vi "read N samples N channels.vi"(8 "error in (no error)":errorcluster, 11 "DAQ  in":refnum<class "DAQ .lvclass">) -> (0 "error out":errorcluster, 2 "data 2":waveform(dbl)[](array[waveform]), 3 "DAQ  out":refnum<class "DAQ .lvclass">)   [LabVIEW 2017, in "Hardware.lvlib" / "DAQ .lvclass"]
uses:
  DAQ .lvclass
  \\Mac\Home/Documents/MAL-Framework/user.lib/Common Components/Hardware/Hardware.lvclass
  DAQ .lvclass/DAQ .ctl
  MAL-Framework/user.lib/Common Components/Hardware/Hardware.lvclass/Hardware.ctl
  <vilib>/DAQmx/read.llb/DAQmx Read (Analog 1D Wfm NChan NSamp).vi
  <vilib>/DAQmx/miscellaneous.llb/DAQmx Fill In Error Info.vi
  MAL-Framework/user.lib/Common Components/Hardware/Hardware.lvclass
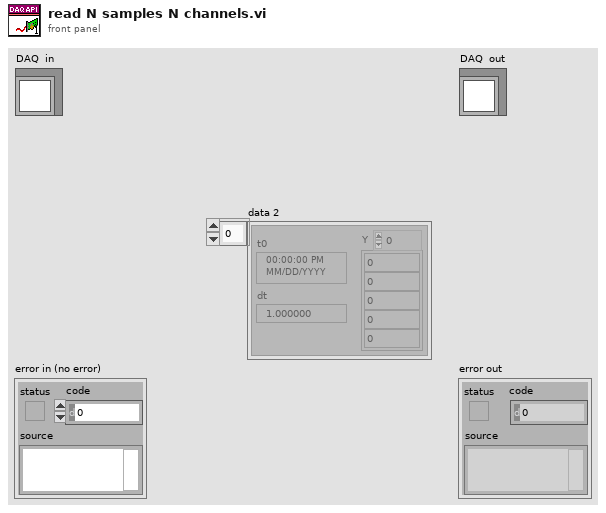
[diagram p1: front panel]
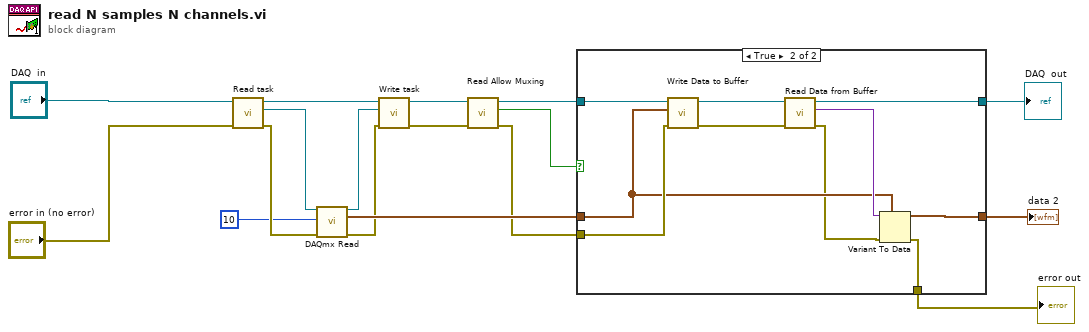
[diagram p0: block diagram]
diagram:
  n1 = call "Read task.vi"("error in (no error)"="error in (no error)", "DAQ  in"="DAQ  in") -> ("error out"=w8:errorcluster, "task"=w15:refnum<k21>, "DAQ  out"=w13:refnum<class "DAQ .lvclass">)  [unwired: 7 in]
  n2 = call-poly <vilib>:"DAQmx Read.vi"("task/channels in"=w15, "number of samples per channel"=10, "error in"=w8) -> ("task out"=w14:refnum<k21>, "data"=w12:waveform(dbl)[], "error out"=w6:errorcluster)  [unwired: 10 in]
  n3 = call "Write task.vi"("error in (no error)"=w6, "task"=w14, "DAQ  in"=w13) -> ("error out"=w7:errorcluster, "DAQ  out"=w11:refnum<class "DAQ .lvclass">)  [unwired: 7 in]
  n4 = call "Read Allow Muxing.vi"("error in (no error)"=w7, "Hardware in"=w11) -> ("error out"=w5:errorcluster, "Allow Muxing"=w9:bool, "Hardware out"=w10:refnum<class "DAQ .lvclass">)  [unwired: 7 in]
  n5 = case shown="True" w9 {
    tunnel: [w19 w29] -> w3
    tunnel: w5 -> [w18 w27]
    tunnel: w12 -> [w20 w25]
    tunnel: [w20 w24] -> w1
    tunnel: [w18 w22] -> w2
    tunnel: w10 -> [w19 w21]
    frame False {
    }
    frame True {
      n6 = call "Write Data to Buffer.vi"("error in (no error)"=w27, "Data"=w25, "Hardware in"=w21) -> ("error out"=w28:errorcluster, "Hardware out"=w30:refnum<class "DAQ .lvclass">)  [unwired: 7 in]
      n7 = call "Read Data from Buffer.vi"("error in (no error)"=w28, "Hardware in"=w30) -> ("error out"=w23:errorcluster, "Variant"=w26:variant, "Hardware out"=w29:refnum<class "DAQ .lvclass">)  [unwired: 7 in]
      n8 = Variant To Data(error in=w23, type=w25, Variant=w26) -> (data=w24:waveform(dbl)[], error out=w22:errorcluster)
    }
  }
  "error out" <- w2
  "DAQ  out" <- w3
  "data 2" <- w1
